vi "Stop Core.vi"(10 "final error code":i32, 11 "UI Main in":refnum<class "UI Main.lvclass">) -> (3 "UI Main out":refnum<class "UI Main.lvclass">)   [LabVIEW 2020, in "UI Main.lvlib" / "UI Main.lvclass"]
doc: "(<B>Filename</B>: Actor Framework.lvlib:Actor.lvclass:Stop Core.vi)\n\nDefines what the actor does before it stops. Use the <B>final error code</B> input to determine whether the actor shut down in response to an error.\n\nBy default, this method passes the Stop message along to all auto-stop nested actors. A descendant class may override this method to define additional behavior, such as shutting down any processes the actor initiated in its override of the Actor Core method."
uses:
  UI Main.lvclass
  UI Main.lvclass/UI Main.ctl
  <vilib>/ActorFramework/Actor/Actor.lvclass
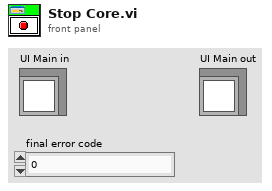
[diagram p1: front panel]
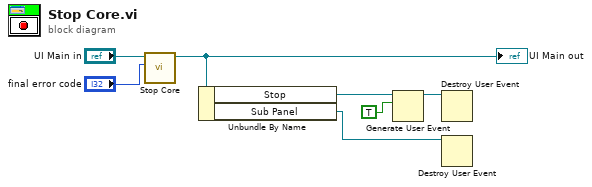
[diagram p0: block diagram]
diagram:
  n1 = call-parent "Stop Core.vi"("final error code"="final error code", "Actor in"="UI Main in") -> ("Actor out"=w5:refnum<class "UI Main.lvclass">)  [unwired: 9 in]
  "UI Main out" <- w5
  n2 = Unbundle By Name(w5) -> ("Stop"=w2:refnum<user-event>, "Sub Panel"=w1:refnum<user-event>)
  n3 = Generate User Event(user event=w2, event data cluster=TRUE ("event data")) -> (user event out=w3:refnum<user-event>)  [unwired: 2 in, 1 out]
  n4 = Destroy User Event(user event=w3) -> ()  [unwired: 1 in, 1 out]
  n5 = Destroy User Event(user event=w1) -> ()  [unwired: 1 in, 1 out]
